vi "Parse Execution Time.vi"(10 "Item":string, 11 "Result Model in":refnum<class "Result Model.lvclass">) -> (3 "Numeric":dbl)   [LabVIEW 2020, in "Result Model Result Recording Test.lvclass"]
uses:
  Result Model Result Recording Test.lvclass
  source/User Interface/Result Model/Result Model.lvclass
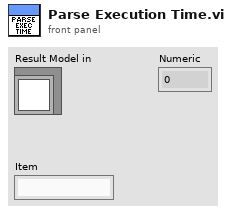
[diagram p1: front panel]
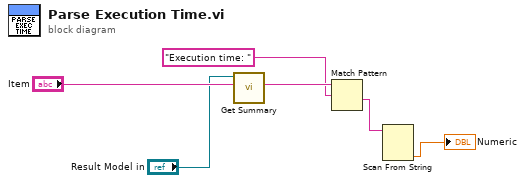
[diagram p0: block diagram]
diagram:
  n1 = call "Get Summary.vi"("Item"="Item", "Result Model by Reference In"="Result Model in") -> ("Summary"=w4:string)  [unwired: 8 in, 1 out]
  n2 = Match Pattern(string=w4, regular expression="Execution time: " ("format string")) -> (after substring=w2:string)  [unwired: 1 in, 3 out]
  n3 = Scan From String(input string=w2) -> (output 1=→"Numeric":dbl)  [unwired: 4 in, 3 out]
